vi "RunVernierCalibV1729A.vi"(4 "# Events to Avg":i32, 6 "# Samples after Trig":u16, 7 "Clock Divisor":u32=2, 8 "error in (no error)":errorcluster, 9 "handle in":i32, 10 "Init State":T2(ring), 11 "VME Base Address in":u32 format="%.0x") -> (0 "error out":errorcluster, 1 "handle out":i32, 2 "Data Out":u32[][](array[numeric]), 3 "Offset":i16)   [LabVIEW 2014]
uses:
  <vilib>/Analysis/baseanly.llb/Mean (DBL).vi
  Program Files (x86)/CAEN/Comm/labview/CAENComm.lvlib
  <vilib>/Analysis/NI_AALBase.lvlib
panel:
  out "Histogram Ch 0 - Ch 3":T1(graph)
  out "Histogram Ch 0 - Ch 2":T1(graph)
  out "Histogram Ch 0 - Ch 1":T1(graph)
  out "mean mean":dbl format="%0.2f"
  out "mean All":dbl format="%0.2f"
  out "mean 3":dbl format="%0.2f"
  out "mean 2":dbl format="%0.2f"
  out "mean 1":dbl format="%0.2f"
  out "mean 0":dbl format="%0.2f"
  out "Histogram Mean":T1(graph)
  out "Histogram Ch 1":T1(graph)
  out "Histogram Ch 3":T1(graph)
  out "Histogram Ch 2":T1(graph)
  out "Histogram Ch 0":T1(graph)
  out "Vernier Data":u16[](array[numeric])
  out "Channel Data":u16[][](array[numeric])
  in  "milliseconds to wait":u32
  out "Histogram Graph":T1(graph)
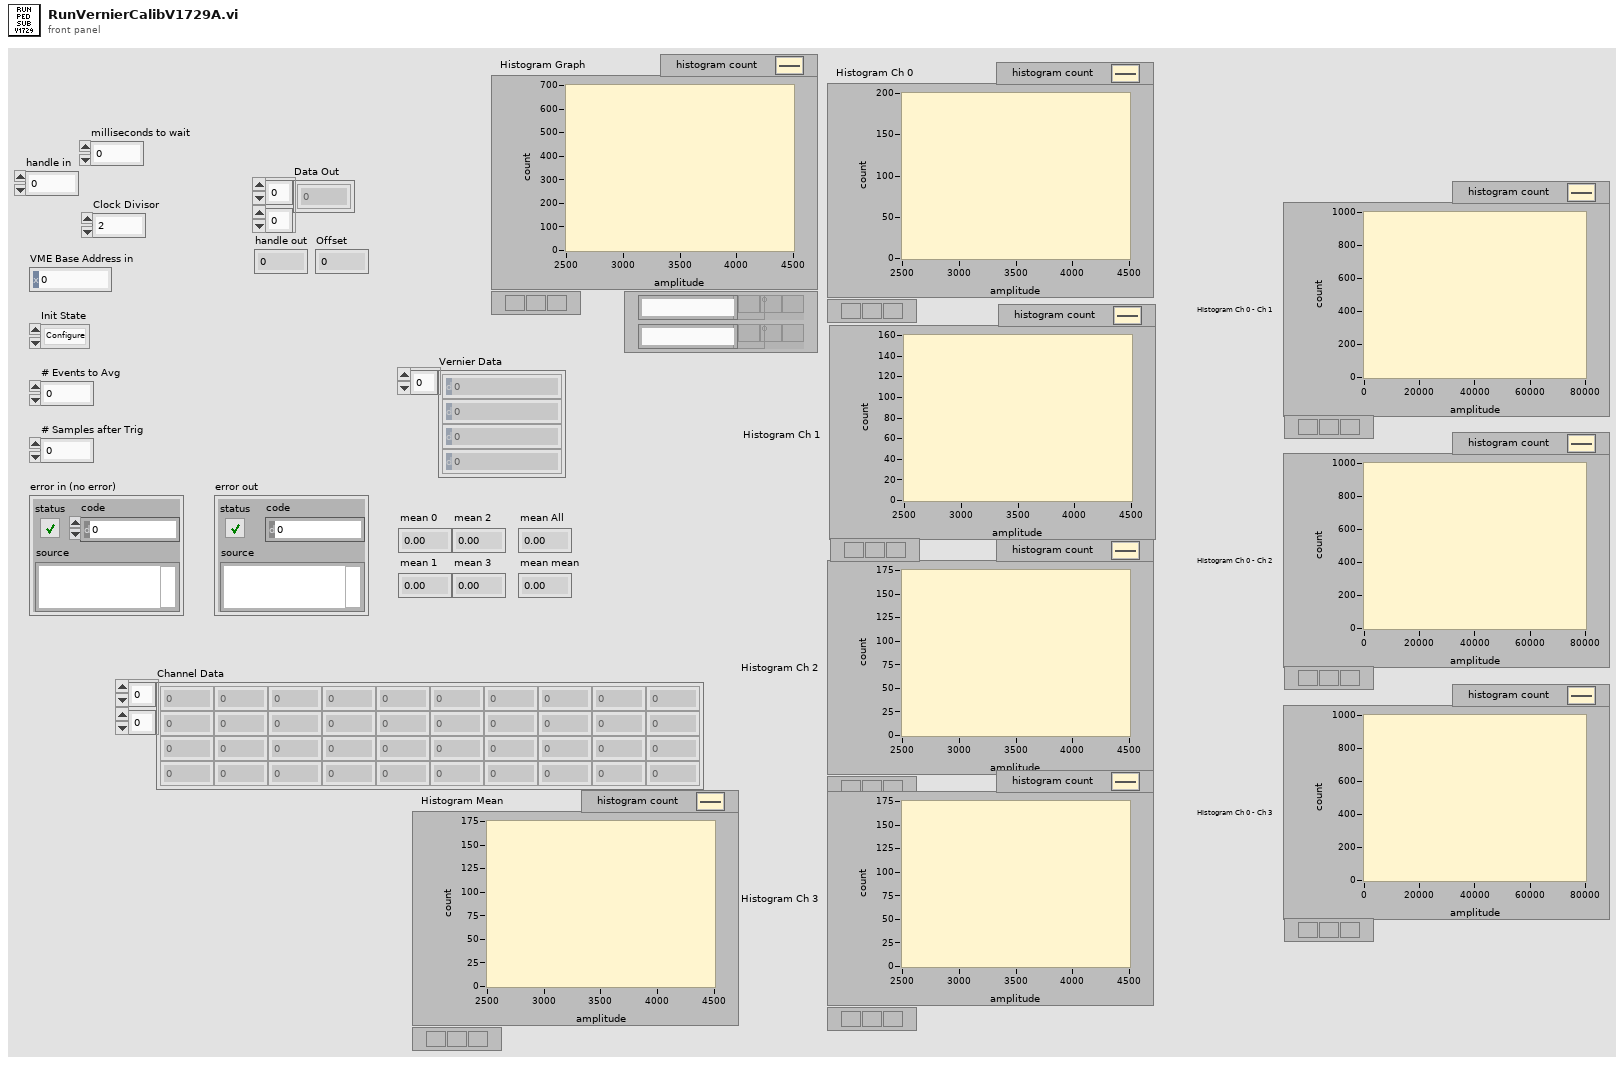
[diagram p1: front panel]
types:
  T1 = cluster{"X Values":dbl[], "Histogram: h(x)":i32[]}
  T2 = enum16{"Configure", "Initialise", "Run", "Close"}
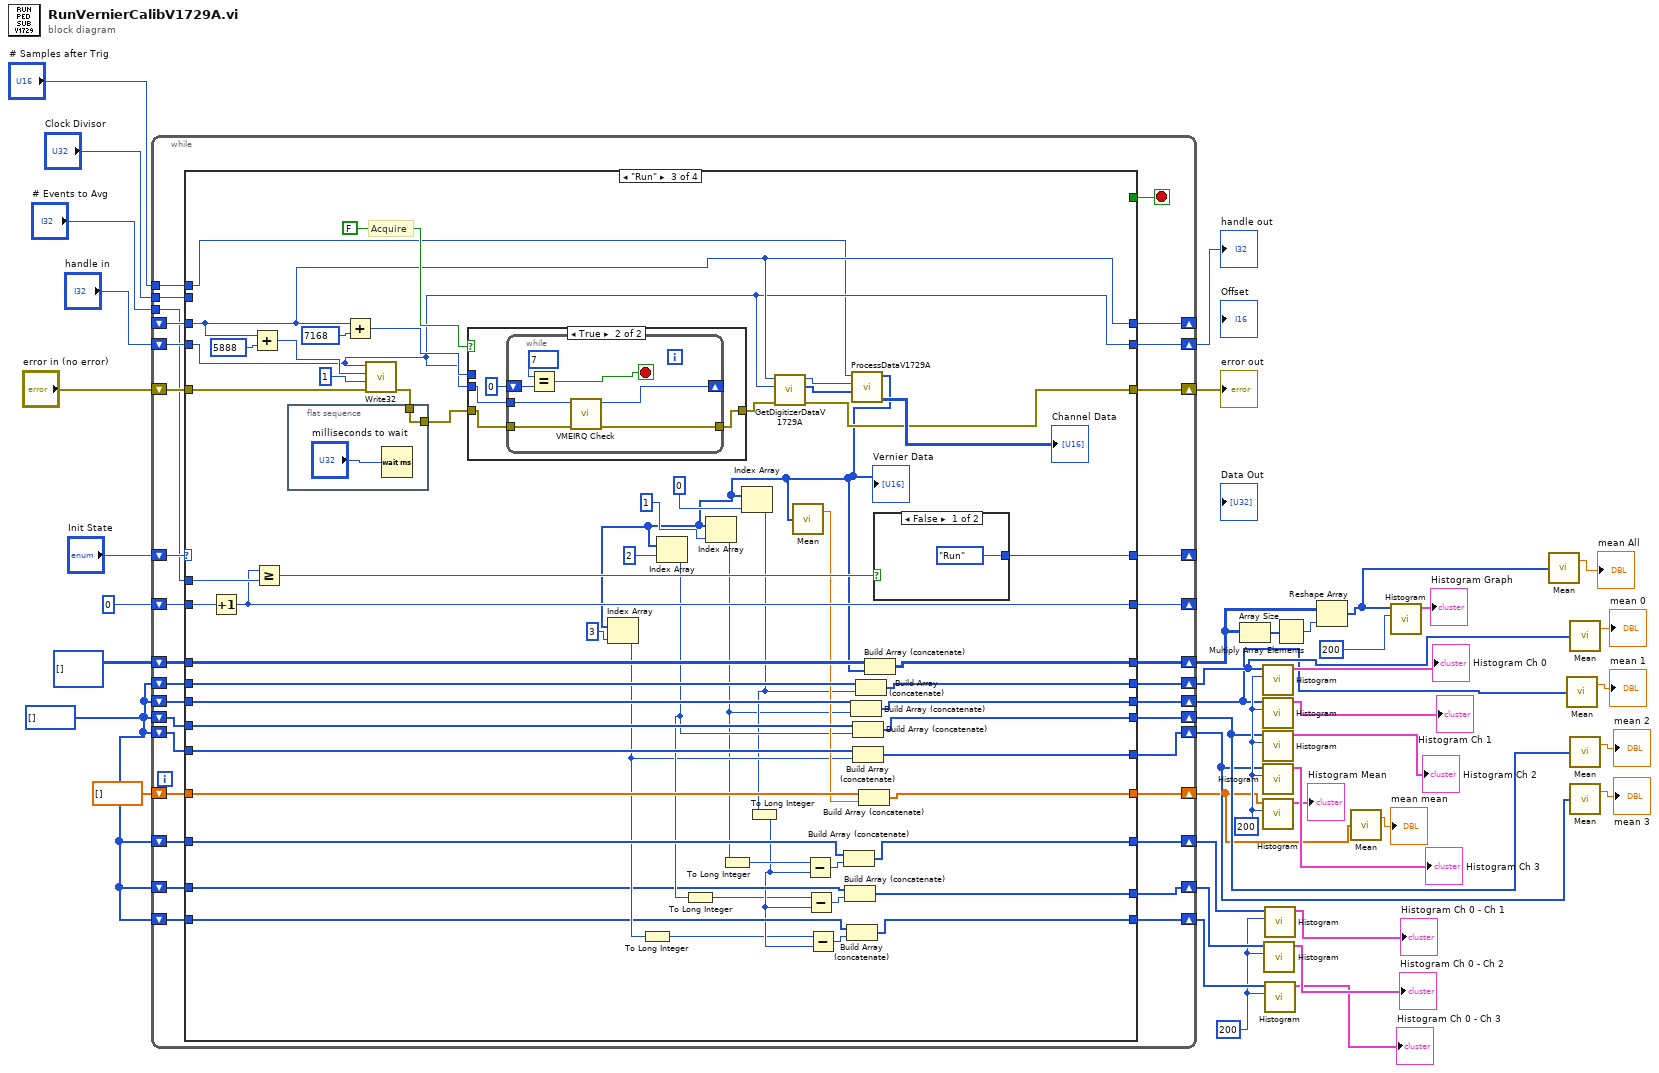
[diagram p0: block diagram]
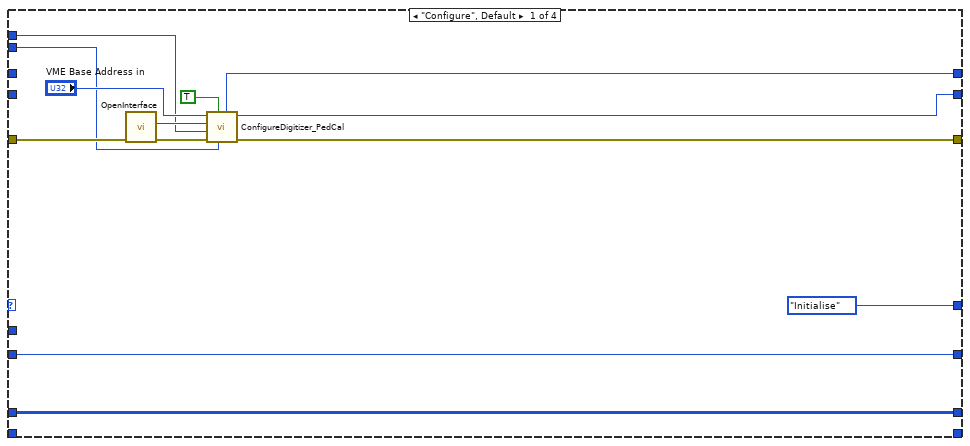
[diagram p2: hidden frame]
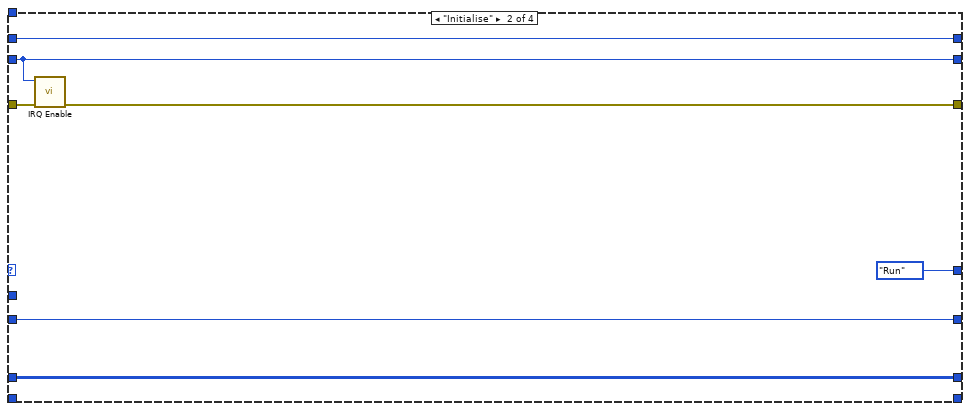
[diagram p3: hidden frame]
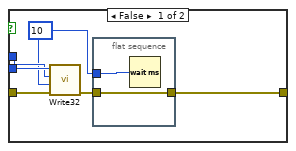
[diagram p4: hidden frame]
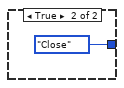
[diagram p5: hidden frame]
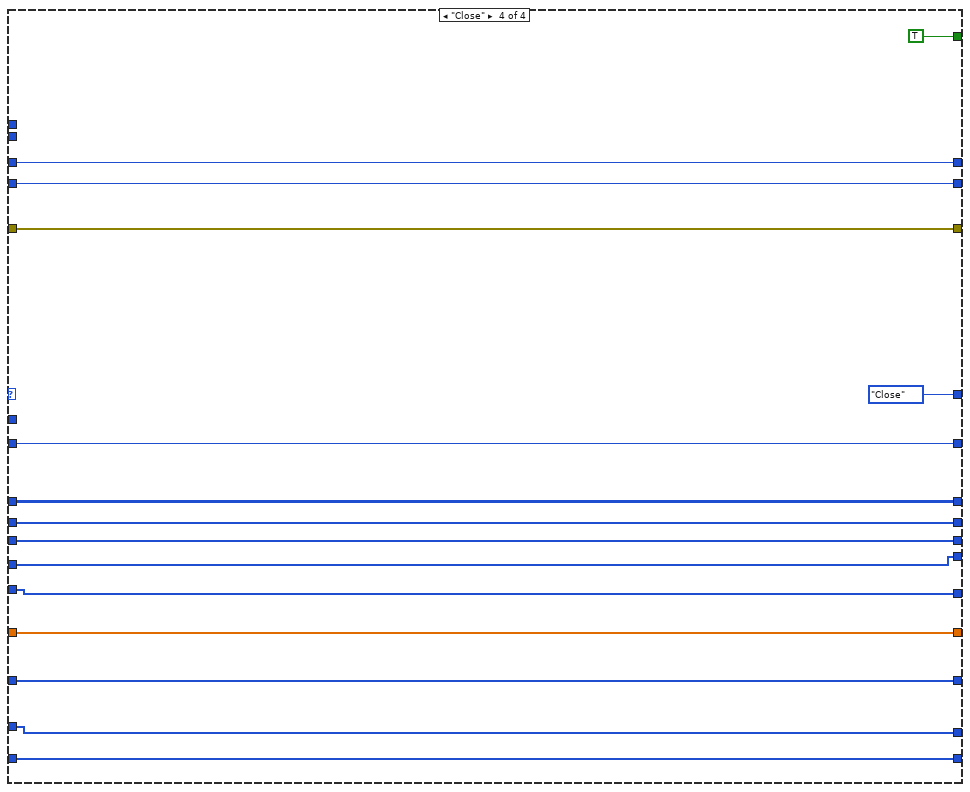
[diagram p6: hidden frame]
diagram:
  w4 = 200 ("samples")
  w22 = 200 ("samples")
  w8 = u16[] [] ("Vernier Data")
  n1 = while {
    shift-right: [w67] -> _
    shift-left: "Init State" -> [w74]
    shift-right: [w72] -> w41
    shift-left: "error in (no error)" -> [w73]
    shift-right: [w71] -> _
    shift-left: _ -> [w68]
    shift-right: [w70] -> w35
    shift-left: "handle in" -> [w69]
    tunnel: "# Events to Avg" -> [w65]
    shift-right: [w63] -> _
    shift-left: 0 -> [w66]
    tunnel: "# Samples after Trig" -> [w62]
    tunnel: "Clock Divisor" -> [w61]
    shift-right: [w59] -> w30
    shift-left: u32[][] [] ("appended array") -> [w60]
    shift-right: [w54] -> w20
    shift-left: w8 -> [w58]
    shift-right: [w53] -> w19
    shift-left: w8 -> [w57]
    shift-right: [w52] -> w18
    shift-left: w8 -> [w56]
    shift-right: [w51] -> w17
    shift-left: w8 -> [w55]
    shift-right: [w49] -> w10
    shift-left: dbl[] [] -> [w50]
    shift-right: [w47] -> w7
    shift-left: w8 -> [w48]
    shift-right: [w44] -> w5
    shift-left: w8 -> [w46]
    shift-right: [w43] -> w6
    shift-left: w8 -> [w45]
    stop <- w64 stop-if-true
    n2 = case shown="\"Run\"" w74 {
      tunnel: w73 -> [w87 w94 w148 w184]
      tunnel: [w84 w89 w128 w184] -> w72
      tunnel: [w81 w92 w134 w187] -> w71
      tunnel: [w80 w93 w133 w188] -> w70
      tunnel: w69 -> [_ w93 w133 w188]
      tunnel: w68 -> [_ w92 w134 w187]
      tunnel: [T2."Initialise" T2."Run" w147 T2."Close"] -> w67
      tunnel: w66 -> [w78 w90 w146 w185]
      tunnel: w65 -> [_ _ w145 _]
      tunnel: [_ _ _ TRUE] -> w64
      tunnel: [w78 w90 w144 w185] -> w63
      tunnel: w62 -> [w77 _ w132 _]
      tunnel: w61 -> [w76 _ _ _]
      tunnel: w60 -> [w75 w88 w139 w183]
      tunnel: [w75 w88 w138 w183] -> w59
      tunnel: w58 -> [_ _ w123 w182]
      tunnel: w57 -> [_ _ w122 w181]
      tunnel: w56 -> [_ _ w121 w180]
      tunnel: w55 -> [_ _ w120 w179]
      tunnel: [_ _ w119 w182] -> w54
      tunnel: [_ _ w118 w181] -> w53
      tunnel: [_ _ w117 w180] -> w52
      tunnel: [_ _ w116 w179] -> w51
      tunnel: w50 -> [_ _ w115 w178]
      tunnel: [_ _ w114 w178] -> w49
      tunnel: w48 -> [_ _ w110 w177]
      tunnel: [_ _ w109 w177] -> w47
      tunnel: w46 -> [_ _ w103 w176]
      tunnel: w45 -> [_ _ w102 w175]
      tunnel: [_ _ w101 w176] -> w44
      tunnel: [_ _ w100 w175] -> w43
      frame "Configure", Default {
        n3 = call "OpenInterface.vi"("error in (no error)"=w87) -> ("error out"=w86:errorcluster, "handle"=w85:i32)  [unwired: 8 in, 1 out]
        n4 = call "ConfigureDigitizer_PedCal.vi"("Clock Divisor"=w76, "Software Trig?"=TRUE, "error in (no error)"=w86, "# Samples after Trig"=w77, "handle"=w85, "VME Base Address"="VME Base Address in") -> ("error out"=w84:errorcluster, "handle out"=w80:i32, "VME Base Address out"=w81:u32)  [unwired: 3 in]
      }
      frame "Initialise" {
        n5 = call "IRQ Enable.vi"("error in (no error)"=w94, "handle"=w93) -> ("error out"=w89:errorcluster)  [unwired: 9 in]
      }
      frame "Run" {
        # "Acquire"
        n6 = Increment(x=w146) -> (x+1=w144:i32)
        n7 = Add(x=w134, y=u32 5888 ("x")) -> (x+y=w150:u32)
        n8 = Greater Or Equal?(x=w144, y=w145) -> (x >= y?=w143:bool)
        n9 = flat-sequence {
          tunnel: w137 -> [w152]
          tunnel: [w152] -> w136
          frame #0 {
            n10 = Wait (ms)(milliseconds to wait="milliseconds to wait") -> ()  [unwired: 1 out]
          }
        }
        n11 = Add(x=w134, y=u32 7168 ("x")) -> (x+y=w140:u32)
        n12 = call "Write32.vi"("error in (no error)"=w148, "Data"=u32 1, "Address"=w150, "handle"=w133) -> ("error out"=w137:errorcluster)  [unwired: 7 in]
        n13 = case shown="True" FALSE {
          tunnel: w136 -> [w157 w164]
          tunnel: [w154 w162] -> w135
          tunnel: w133 -> [w159 w165]
          tunnel: w140 -> [w158 _]
          frame False {
            w156 = u32 10 ("Data")
            n14 = call "Write32.vi"("error in (no error)"=w157, "Data"=w156, "Address"=w158, "handle"=w159) -> ("error out"=w155:errorcluster)  [unwired: 7 in]
            n15 = flat-sequence {
              tunnel: w156 -> [w160]
              tunnel: w155 -> [w161]
              tunnel: [w161] -> w154
              frame #0 {
                n16 = Wait (ms)(milliseconds to wait=w160) -> ()  [unwired: 1 out]
              }
            }
          }
          frame True {
            n17 = while {
              tunnel: [w169] -> w162
              tunnel: w165 -> [w172]
              shift-right: [w171] -> _
              shift-left: u8 0 ("Mask") -> [w168]
              tunnel: w164 -> [w170]
              stop <- w166 stop-if-true
              n18 = Equal?(x=u8 7 ("y"), y=w168) -> (x = y?=w166:bool)
              n19 = call "VMEIRQ Check.vi"("error in (no error)"=w170, "VMEhandle"=w172) -> ("error out"=w169:errorcluster, "Mask"=w171:u8)  [unwired: 8 in]
            }
          }
        }
        n20 = call "GetDigitizerDataV1729A.vi"("error in (no error)"=w135, "handle in"=w133, "VME Base Address"=w134) -> ("error out"=w128:errorcluster, "Waveform"=w130:u32[], "TRIG_REC"=w131:u32)  [unwired: 4 in, 2 out]
        n21 = call "ProcessDataV1729A.vi"("Buffer"=w130, "TRIG_REC"=w131, "# Samples after Trig"=w132) -> ("Channel Data"=→"Channel Data":u16[][], "Vernier Data"=w113:u16[])  [unwired: 7 in]
        "Vernier Data" <- w113
        n22 = Index Array(array=w113, index=3) -> (element=w105:u16)
        n23 = To Long Integer(number=w105) -> (32bit integer=w95:i32)
        n24 = Index Array(array=w113, index=2) -> (element=w107:u16)
        n25 = To Long Integer(number=w107) -> (32bit integer=w96:i32)
        n26 = Index Array(array=w113, index=1) -> (element=w99:u16)
        n27 = To Long Integer(number=w99) -> (32bit integer=w98:i32)
        n28 = Index Array(array=w113, index=0) -> (element=w104:u16)
        n29 = To Long Integer(number=w104) -> (32bit integer=w97:i32)
        n30 = call-poly <vilib>:"Mean.vi"("X"=w113) -> ("mean"=w112:dbl)  [unwired: 1 out]
        n31 = Subtract(x=w98, y=w97) -> (x-y=w111:i32)
        n32 = Subtract(x=w96, y=w97) -> (x-y=w108:i32)
        n33 = Subtract(x=w95, y=w97) -> (x-y=w106:i32)
        n34 = Build Array (concatenate)(w110, w111) -> (w109:i32[])
        n35 = Build Array (concatenate)(w103, w108) -> (w101:i32[])
        n36 = Build Array (concatenate)(w102, w106) -> (w100:i32[])
        n37 = Build Array (concatenate)(w122, w99) -> (w118:u16[])
        n38 = Build Array (concatenate)(w121, w107) -> (w117:u16[])
        n39 = Build Array (concatenate)(w120, w105) -> (w116:u16[])
        n40 = Build Array (concatenate)(w123, w104) -> (w119:u16[])
        n41 = Build Array (concatenate)(w115, w112) -> (w114:dbl[])
        n42 = Build Array (concatenate)(w139, w113) -> (w138:u32[][])
        n43 = case shown="False" w143 {
          tunnel: [T2."Run" T2."Close"] -> w147
          frame False {
          }
          frame True {
          }
        }
      }
      frame "Close" {
      }
    }
  }
  "error out" <- w41
  "handle out" <- w35
  n44 = Array Size(array=w30) -> (size(s)=w32:i32[])
  n45 = call <vilib>:"Histogram.vi"("intervals"=w22, "X"=w20) -> ("Histogram Graph"=→"Histogram Ch 0":T1)  [unwired: 6 in, 3 out]
  n46 = call <vilib>:"Histogram.vi"("intervals"=w22, "X"=w19) -> ("Histogram Graph"=→"Histogram Ch 1":T1)  [unwired: 6 in, 3 out]
  n47 = call <vilib>:"Histogram.vi"("intervals"=w22, "X"=w18) -> ("Histogram Graph"=→"Histogram Ch 2":T1)  [unwired: 6 in, 3 out]
  n48 = call <vilib>:"Histogram.vi"("intervals"=w22, "X"=w17) -> ("Histogram Graph"=→"Histogram Ch 3":T1)  [unwired: 6 in, 3 out]
  n49 = call <vilib>:"Histogram.vi"("intervals"=w22, "X"=w10) -> ("Histogram Graph"=→"Histogram Mean":T1)  [unwired: 6 in, 3 out]
  n50 = call <vilib>:"Histogram.vi"("intervals"=w4, "X"=w5) -> ("Histogram Graph"=→"Histogram Ch 0 - Ch 2":T1)  [unwired: 6 in, 3 out]
  n51 = call <vilib>:"Histogram.vi"("intervals"=w4, "X"=w7) -> ("Histogram Graph"=→"Histogram Ch 0 - Ch 1":T1)  [unwired: 6 in, 3 out]
  n52 = call <vilib>:"Histogram.vi"("intervals"=w4, "X"=w6) -> ("Histogram Graph"=→"Histogram Ch 0 - Ch 3":T1)  [unwired: 6 in, 3 out]
  n53 = Multiply Array Elements(1:w32) -> (0:w31:i32)
  n54 = Reshape Array(w30, w31) -> (w12:u32[])
  n55 = call-poly <vilib>:"Mean.vi"("X"=w10) -> ("mean"=→"mean mean":dbl)  [unwired: 1 out]
  n56 = call <vilib>:"Histogram.vi"("intervals"=200 ("samples"), "X"=w12) -> ("Histogram Graph"=→"Histogram Graph":T1)  [unwired: 6 in, 3 out]
  n57 = call-poly <vilib>:"Mean.vi"("X"=w12) -> ("mean"=→"mean All":dbl)  [unwired: 1 out]
  n58 = call-poly <vilib>:"Mean.vi"("X"=w19) -> ("mean"=→"mean 1":dbl)  [unwired: 1 out]
  n59 = call-poly <vilib>:"Mean.vi"("X"=w20) -> ("mean"=→"mean 0":dbl)  [unwired: 1 out]
  n60 = call-poly <vilib>:"Mean.vi"("X"=w18) -> ("mean"=→"mean 2":dbl)  [unwired: 1 out]
  n61 = call-poly <vilib>:"Mean.vi"("X"=w17) -> ("mean"=→"mean 3":dbl)  [unwired: 1 out]
